vi "Grade VI Results.vi"(8 "Error in":errorcluster caption="Error in (no error)", 11 "VIAResult":T11 {"Test Config Data"."Test Ranking" items=["Low", "Normal", "High"]}) -> (0 "Error out":errorcluster, 3 "VI Stats Map":map{path, T1}(c390))   [LabVIEW 2023, in "VIA Results Handling.lvlib"]
doc: "Converts VIA Results data into a VI Stats Map"
uses:
  VIA Results Handling.lvlib
  <vilib>/addons/analyzer/_analyzerctrls.llb/VIAnCtl Results.ctl
  <vilib>/addons/analyzer/_analyzerctrls.llb/VIAnCtl ResultsData (index).ctl
  <vilib>/addons/analyzer/_analyzerctrls.llb/VIAnCtl ResultStatus.ctl
  <vilib>/addons/analyzer/_vianresshared.llb/VIAnRes Parsed Results Data (by VI).ctl
  <vilib>/addons/analyzer/_vianresshared.llb/VIAnRes Parsed Results Data (by Test).ctl
  <vilib>/addons/analyzer/_analyzerctrls.llb/VIAnCtl Test Config Data.ctl
  <vilib>/addons/analyzer/_analyzerctrls.llb/VIAnCtl TestRanking.ctl
  <vilib>/addons/analyzer/_analyzerctrls.llb/VIAnCtl Config Control Value.ctl
  Stats by Ranking.ctl
  Stats Cluster.ctl
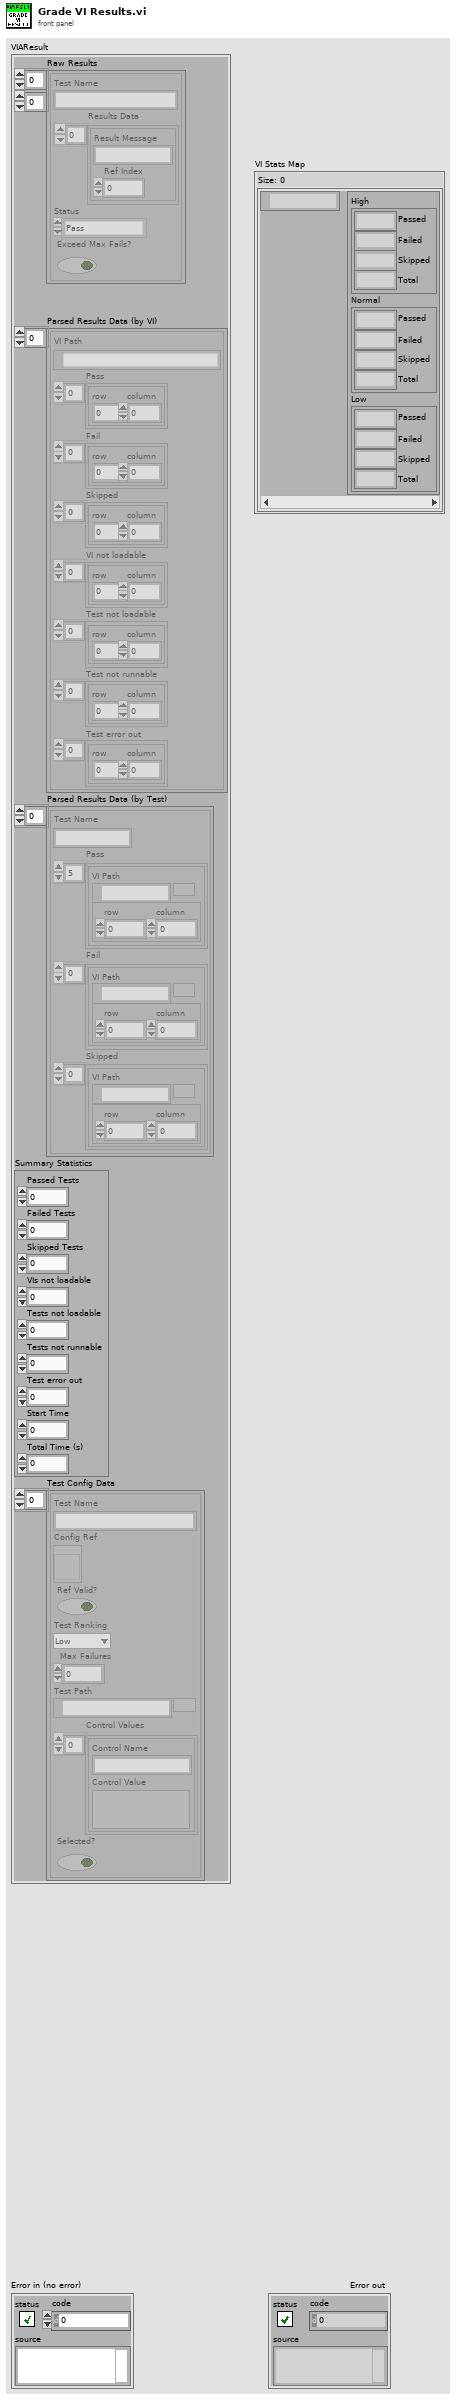
[diagram p1: front panel]
types:
  T1 = typedef "VIA Results Handling.lvlib/Stats by Ranking.ctl" = cluster{"High":T2, "Normal":T2, "Low":T2}
  T2 = typedef "VIA Results Handling.lvlib/Stats Cluster.ctl" = cluster{"Passed":i32, "Failed":i32, "Skipped":i32, "Total":i32}
  T3 = typedef "VIAnCtl Results.ctl" = cluster{"Test Name":string, "Results Data":T4[], "Status":T5, "Exceed Max Fails?":bool}
  T4 = typedef "VIAnCtl ResultsData (index).ctl" = cluster{"Result Message":string, "Ref Index":i32}
  T5 = typedef "VIAnCtl ResultStatus.ctl" = enum16{"Pass", "Fail", "Skipped", "VI not loadable", "Test not loadable", "Test not runnable", "Test error out"}
  T6 = typedef "VIAnRes Parsed Results Data (by VI).ctl" = cluster{"VI Path":path, "Pass":cluster{"row":i32, "column":i32}[], "Fail":cluster{"row":i32, "column":i32}[], "Skipped":cluster{"row":i32, "column":i32}[], "VI not loadable":cluster{"row":i32, "column":i32}[], "Test not loadable":cluster{"row":i32, "column":i32}[], "Test not runnable":cluster{"row":i32, "column":i32}[], "Test error out":cluster{"row":i32, "column":i32}[]}
  T7 = typedef "VIAnRes Parsed Results Data (by Test).ctl" = cluster{"Test Name":string, "Pass":cluster{"VI Path":path, "index":cluster{"row":i32, "column":i32}}[], "Fail":cluster{"VI Path":path, "index":cluster{"row":i32, "column":i32}}[], "Skipped":cluster{"VI Path":path, "index":cluster{"row":i32, "column":i32}}[]}
  T8 = typedef "VIAnCtl Test Config Data.ctl" = cluster{"Test Name":string, "Config Ref":refnum<vi>, "Ref Valid?":bool, "Test Ranking":T9, "Max Failures":u32, "Test Path":path, "Control Values":T10[], "Selected?":bool}
  T9 = typedef "VIAnCtl TestRanking.ctl" = u16
  T10 = typedef "VIAnCtl Config Control Value.ctl" = cluster{"Control Name":string, "Control Value":variant}
  T11 = cluster{"Raw Results":T3[][], "Parsed Results Data (by VI)":T6[], "Parsed Results Data (by Test)":T7[], "Summary Statistics":cluster{"Passed Tests":i32, "Failed Tests":i32, "Skipped Tests":i32, "VIs not loadable":i32, "Tests not loadable":i32, "Tests not runnable":i32, "Test error out":i32, "Start Time":u32, "Total Time (s)":dbl}, "Test Config Data":T8[]}
  T12 = typedef "VIA Results Handling.lvlib/Test Config Map.ctl" = map{string, T8}
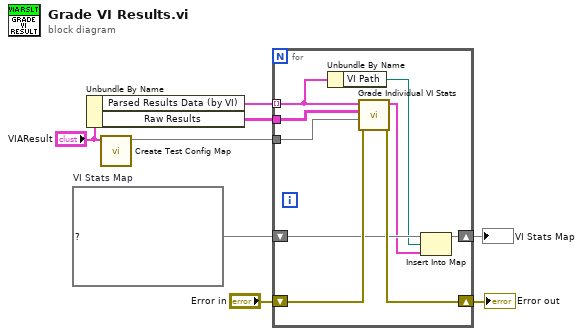
[diagram p0: block diagram]
diagram:
  w2 = map{path, T1} {}  # VI Stats Map
  n1 = Unbundle By Name("VIAResult") -> ("Parsed Results Data (by VI)"=w6:T6[], "Raw Results"=w5:T3[][])
  n2 = call "Create Test Config Map.vi"("VIAResult"="VIAResult") -> ("Test Config Map"=w7:T12)  [unwired: 10 in]
  n3 = for {
    tunnel: w7 -> [w15]
    tunnel: w6 -> [w17] mode=indexing
    tunnel: w5 -> [w16]
    shift-right: [w13] -> w3
    shift-left: "Error in" -> [w14]
    shift-right: [w11] -> w1
    shift-left: w2 -> [w12]
    n4 = Unbundle By Name(w17) -> ("VI Path"=w10:path)
    n5 = call "Grade Individual VI Stats.vi"("Error in"=w14, "Test Config Map"=w15, "Raw Results"=w16, "VI Results"=w17) -> ("Error out"=w13:errorcluster, "Stats by Ranking"=w9:T1)  [unwired: 6 in]
    n6 = Insert Into Map(map in=w12, key=w10, value=w9) -> (map out=w11:map{path, T1})  [unwired: 2 out]
  }
  "Error out" <- w3
  "VI Stats Map" <- w1
